vi "Main Page.vi"(8 "error in (no error)":errorcluster, 11 "Node Ptr":T2 format="%.0x") -> (0 "error out":errorcluster)   [LabVIEW 2017, in "OPC UA Client System Explorer.lvlib"]
uses:
  OPC UA Client System Explorer.lvlib
  <vilib>/NI Veristand/Custom Device API/Custom Device Item Ref.ctl
  Shared/OPCConnection.Properties.ctl
  Shared/Constants.vi
  <vilib>/NI Veristand/Custom Device API/NI VeriStand - Get Item Property.vi
  <vilib>/NI Veristand/Custom Device API/Get Item Property (String).vi
  <vilib>/NI Veristand/Custom Device API/Get Item Property (U16).vi
  <vilib>/NI Veristand/Custom Device API/Get Item Property (Dependent File).vi
  <vilib>/NI Veristand/Custom Device API/NI VeriStand - Set Item Property.vi
  <vilib>/NI Veristand/Custom Device API/Set Item Property (String).vi
  <vilib>/NI Veristand/Custom Device API/Set Item Property (U16).vi
  <vilib>/Utility/libraryn.llb/Get File Extension.vi
  <vilib>/Utility/MD5Checksum.llb/MD5Checksum File.vi
  <vilib>/NI Veristand/Custom Device API/Set Item Property (Dependent File).vi
  <vilib>/NI Veristand/Custom Device API/NI VeriStand - Remove Item Property.vi
  <vilib>/NI VeriStand/Custom Device API/Custom Device API.lvlib
  Shared/OPC UA Client Shared.lvlib
panel:
  in  "Header 2":cluster{"Section Name":string}={"Section Name"="Connection Settings"}
  in  "Login Info":cluster{"User Name":string, "Password":string}
  in  "Security Policy":T1
  in  "Server Certificate":path
  in  "Client Certificate":path
  in  "Server Port":u16=49350
  in  "Server IP Address":string
  in  "SHDocVw.IWebBrowser":refnum<k7>(container)
  in  "Header":cluster{"Section Name":string}={"Section Name"="Custom Device Item Settings"}
  in  "Description":string
  in  "Name":string
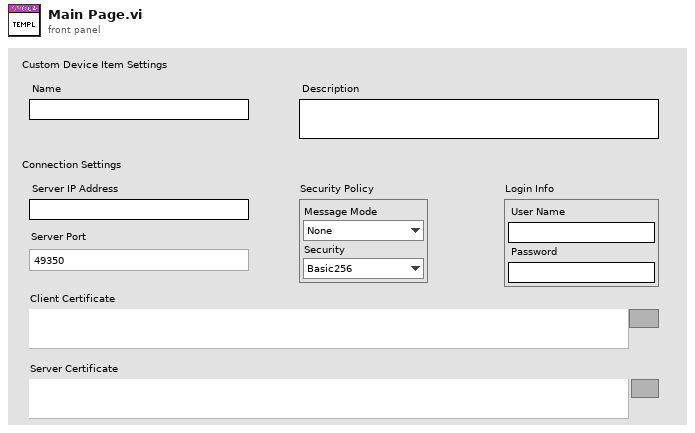
[diagram p1: front panel]
types:
  T1 = cluster{"Message Mode":enum16{"None", "Sign", "Sign and Encrypt"}, "Security":enum16{"Basic256", "Basic128Rsa15"}}
  T2 = typedef "Custom Device API.lvlib/Custom Device Item Ref.ctl" = u64
  T3 = typedef "Custom Device API.lvlib/Custom Device Item Info.ctl" = cluster{"Name":string, "Is Channel":bool, "GUID":string, "Is Waveform":bool}
  T4 = typedef "OPC UA Client Shared.lvlib/OPCConnection.Properties.ctl" = cluster{"Server IP Address":string, "Server Port":u16, "Message Mode":enum16{"None", "Sign", "Sign and Encrypt"}, "Security":enum16{"Basic256", "Basic128Rsa15"}, "User Name":string, "Password":string, "Client Certificate":path, "Server Certificate":path, "Server Certificate (RT)":path, "Client Certificate (RT)":path}
  T5 = typedef "Custom Device API.lvlib/Custom Device Commands.ctl" = enum16{"Default", "Item renamed", "Shutdown", "Dynamic button pressed"}
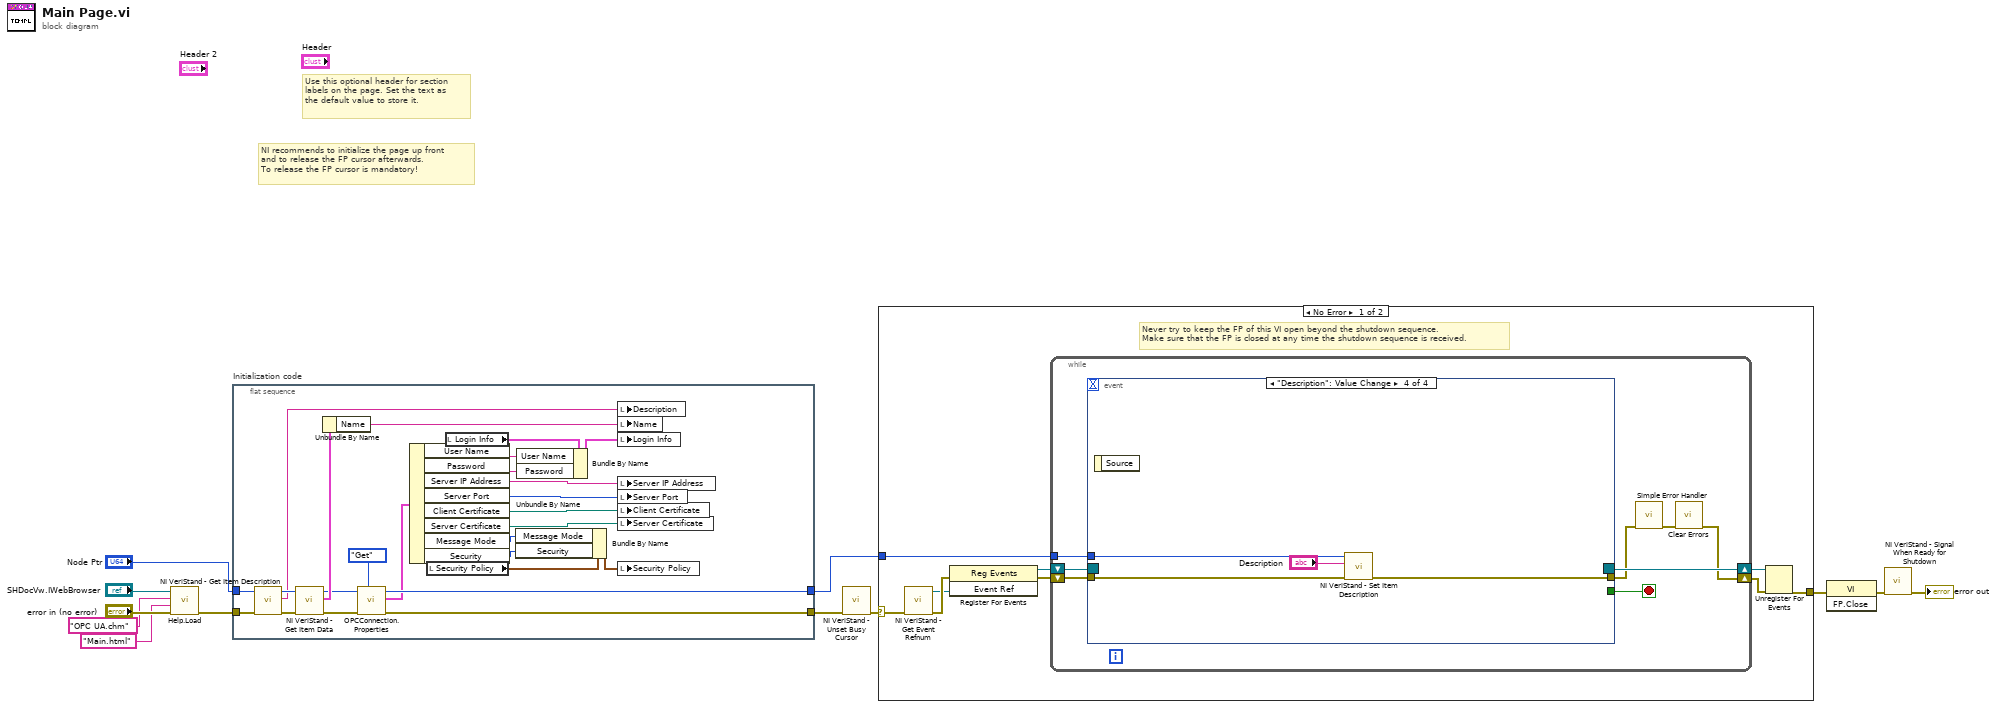
[diagram p0: block diagram]
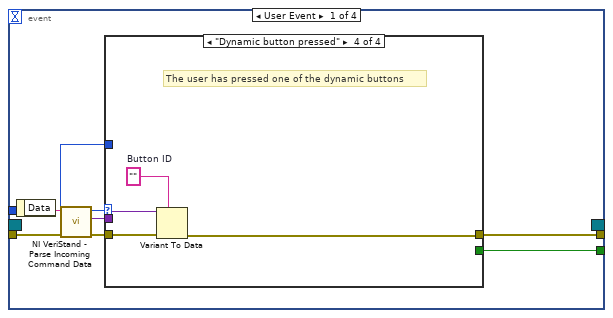
[diagram p2: hidden frame]
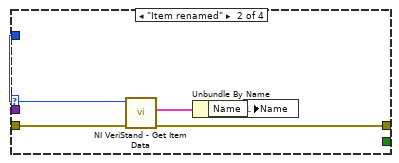
[diagram p4: hidden frame]
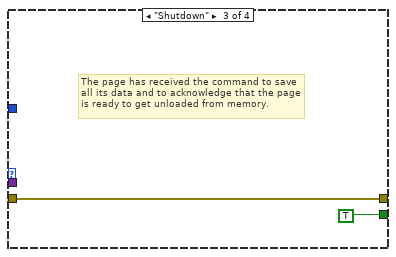
[diagram p5: hidden frame]
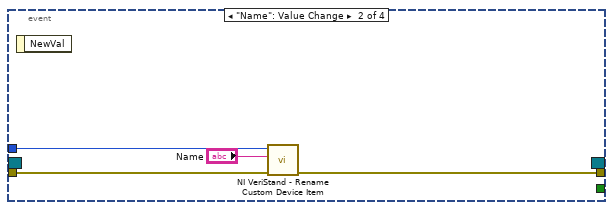
[diagram p6: hidden frame]
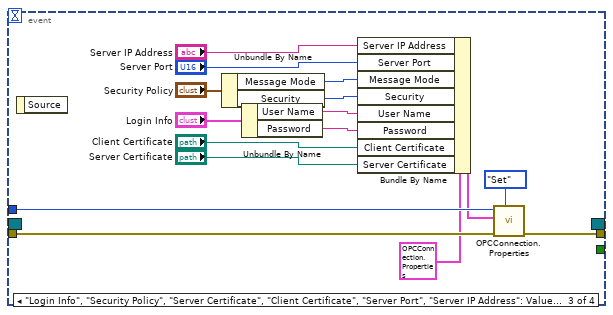
[diagram p7: hidden frame]
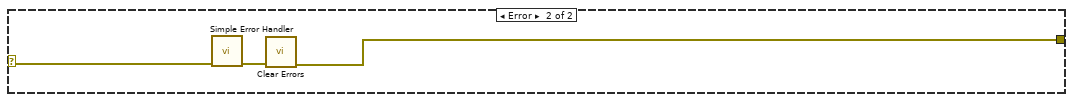
[diagram p8: hidden frame]
diagram:
  # "Use this optional header for section labels on the page. Set the text as the default value to store it."
  # "NI recommends to initialize the page up front\nand to release the FP cursor afterwards.\nTo release the FP cursor is mandatory!"
  n1 = call "Help.Load.vi"("error in (no error)"="error in (no error)", "HTML File"="Main.html" ("Main CHM File"), "Main CHM File"="OPC UA.chm", "SHDocVw.IWebBrowser2"="SHDocVw.IWebBrowser") -> ("error out"=w4:errorcluster)  [unwired: 7 in]
  n2 = flat-sequence "Initialization code" {
    tunnel: w4 -> [w36]
    tunnel: "Node Ptr" -> [w35]
    tunnel: [w28] -> w8
    tunnel: [w26] -> w6
    frame #0 {
      n3 = call <vilib>:"NI VeriStand - Get Item Description.vi"("error in (no error)"=w36, "Item Ref in"=w35) -> ("error out"=w33:errorcluster, "Description"=w34:string, "Item Ref out"=w37:T2)  [unwired: 7 out]
      n4 = call <vilib>:"NI VeriStand - Get Item Data.vi"("error in (no error)"=w33, "Item Ref in"=w37) -> ("error out"=w29:errorcluster, "Item Info"=w32:T3, "Item Ref out"=w27:T2)  [unwired: 7 out]
      n5 = Unbundle By Name(w32) -> ("Name"=w31:string)
      n6 = call "OPCConnection.Properties.vi"("Action"=enum8{"Get", "Set"}."Get", "error in (no error)"=w29, "Item Ref in"=w27) -> ("error out"=w28:errorcluster, "Connection.Properties"=w25:T4, "Item Ref out"=w26:T2)  [unwired: 6 in]
      n7 = Unbundle By Name(w25) -> ("User Name"=w23:string, "Password"=w22:string, "Server IP Address"=w20:string, "Server Port"=w19:u16, "Client Certificate"=w18:path, "Server Certificate"=w17:path, "Message Mode"=w14:enum16{"None", "Sign", "Sign and Encrypt"}, "Security"=w13:enum16{"Basic256", "Basic128Rsa15"})
      n8 = local read "Security Policy"() -> (w15:T1)
      n9 = local read "Login Info"() -> (w24:cluster{"User Name":string, "Password":string})
      n10 = Bundle By Name(cluster=w15, "Message Mode"=w14, "Security"=w13) -> (w16:T1)
      n11 = Bundle By Name(cluster=w24, "User Name"=w23, "Password"=w22) -> (w21:cluster{"User Name":string, "Password":string})
      n12 = local write "Description"(w34) -> ()
      n13 = local write "Name"(w31) -> ()
      n14 = local write "Login Info"(w21) -> ()
      n15 = local write "Server IP Address"(w20) -> ()
      n16 = local write "Server Port"(w19) -> ()
      n17 = local write "Client Certificate"(w18) -> ()
      n18 = local write "Server Certificate"(w17) -> ()
      n19 = local write "Security Policy"(w16) -> ()
    }
  }
  n20 = call <vilib>:"NI VeriStand - Unset Busy Cursor.vi"("error in (no error)"=w8) -> ("error out"=w7:errorcluster)  [unwired: 10 out]
  n21 = case shown="No Error" w7 {
    selector: w7 -> [w38 w101]
    tunnel: [w43 w99] -> w12
    tunnel: w6 -> [w39 _]
    frame No Error {
      # "Never try to keep the FP of this VI open beyond the shutdown sequence.\nMake sure that the FP is closed at any time the shutdown sequence is received."
      n22 = call <vilib>:"NI VeriStand - Get Event Refnum.vi"("error in (no error)"=w38) -> ("error out"=w46:errorcluster, "Event Ref"=w42:refnum<user-event>)  [unwired: 9 out]
      n23 = register-events(error in=w46, w42) -> (reference out=w40:refnum<event-registration>, error out=w41:errorcluster)  [unwired: 1 in]
      n24 = while {
        tunnel: w39 -> [w50]
        shift-right: [w47] -> w44
        shift-left: w41 -> [w53]
        shift-right: [w54] -> w45
        shift-left: w40 -> [w52]
        stop <- w51 stop-if-true
        n25 = event shown="[3] \"Description\": Value Change" {
          selector: w52 -> [_ _ _ _]
          dyn-events: [_ _ _ _] -> w54
          timeout: _ -> [_ _ _ _]
          tunnel: w53 -> [w62 w78 w93 w97]
          tunnel: [w58 _ _ _] -> w51
          tunnel: [w57 w77 w92 w96] -> w49
          tunnel: w50 -> [w56 w76 w91 w98]
          event User Event {
            n26 = event-data() -> ("Data"=w61:string)  [unwired: 1 out]
            n27 = call <vilib>:"NI VeriStand - Parse Incoming Command Data.vi"("error in (no error)"=w62, "Incoming data"=w61) -> ("error out"=w60:errorcluster, "Outgoing data"=w55:variant, "Action"=w59:T5)  [unwired: 7 out]
            n28 = case shown="\"Dynamic button pressed\"" w59 {
              tunnel: w60 -> [w63 w68 w69 w74]
              tunnel: [_ _ TRUE _] -> w58
              tunnel: [w63 w65 w69 w71] -> w57
              tunnel: w56 -> [_ w67 _ _]
              tunnel: w55 -> [_ _ _ w73]
              frame "Default", Default {
              }
              frame "Item renamed" {
                n29 = call <vilib>:"NI VeriStand - Get Item Data.vi"("error in (no error)"=w68, "Item Ref in"=w67) -> ("error out"=w65:errorcluster, "Item Info"=w66:T3)  [unwired: 8 out]
                n30 = Unbundle By Name(w66) -> ("Name"=w64:string)
                n31 = local write "Name"(w64) -> ()
              }
              frame "Shutdown" {
                # "The page has received the command to save all its data and to acknowledge that the page is ready to get unloaded from memory."
              }
              frame "Dynamic button pressed" {
                w72 = ""  # Button ID
                # "The user has pressed one of the dynamic buttons"
                n32 = Variant To Data(error in=w74, type=w72, Variant=w73) -> (error out=w71:errorcluster)  [unwired: 1 out]
              }
            }
          }
          event "Name": Value Change {
            n33 = event-data() -> ()  [unwired: 2 out]
            n34 = call <vilib>:"NI VeriStand - Rename Custom Device Item.vi"("error in (no error)"=w78, "New Name"="Name", "Item Ref in"=w76) -> ("error out"=w77:errorcluster)  [unwired: 1 in, 7 out]
          }
          event "Login Info", "Security Policy", "Server Certificate", "Client Certificate", "Server Port", "Server IP Address": Value Change {
            n35 = event-data() -> ()  [unwired: 2 out]
            n36 = Unbundle By Name("Security Policy") -> ("Message Mode"=w83:enum16{"None", "Sign", "Sign and Encrypt"}, "Security"=w82:enum16{"Basic256", "Basic128Rsa15"})
            n37 = Unbundle By Name("Login Info") -> ("User Name"=w86:string, "Password"=w85:string)
            n38 = Bundle By Name(cluster=T4 {"Server IP Address"="localhost", "Server Port"=49350, "Message Mode"=enum."None", "Security"=enum."Basic256", "User Name"="", "Password"="", "Client Certificate"=path "", "Server Certificate"=path "", "Server Certificate (RT)"=path "", "Client Certificate (RT)"=path ""} ("Connection.Properties"), "Server IP Address"="Server IP Address", "Server Port"="Server Port", "Message Mode"=w83, "Security"=w82, "User Name"=w86, "Password"=w85, "Client Certificate"="Client Certificate", "Server Certificate"="Server Certificate") -> (w79:T4)
            n39 = call "OPCConnection.Properties.vi"("Action"=enum8{"Get", "Set"}."Set", "error in (no error)"=w93, "Connection.Properties"=w79, "Item Ref in"=w91) -> ("error out"=w92:errorcluster)  [unwired: 5 in, 2 out]
          }
          event "Description": Value Change {
            n40 = event-data() -> ()  [unwired: 2 out]
            n41 = call <vilib>:"NI VeriStand - Set Item Description.vi"("error in (no error)"=w97, "Description"="Description", "Item Ref in"=w98) -> ("error out"=w96:errorcluster)  [unwired: 8 out]
          }
        }
        n42 = call <vilib>:"Simple Error Handler.vi"("error in (no error)"=w49) -> ("error out"=w48:errorcluster)  [unwired: 1 in, 7 out]
        n43 = call <vilib>:"Clear Errors.vi"("error in (no error)"=w48) -> ("error out"=w47:errorcluster)  [unwired: 1 in, 5 out]
      }
      n44 = Unregister For Events(event registration refnum=w45, error in=w44) -> (error out=w43:errorcluster)
    }
    frame Error {
      n45 = call <vilib>:"Simple Error Handler.vi"("error in (no error)"=w101) -> ("error out"=w100:errorcluster)  [unwired: 1 in, 7 out]
      n46 = call <vilib>:"Clear Errors.vi"("error in (no error)"=w100) -> ("error out"=w99:errorcluster)  [unwired: 1 in, 5 out]
    }
  }
  n47 = invoke class="VI" method="FP.Close"(error in=w12) -> (error out=w11:errorcluster)  [unwired: 2 in, 2 out]
  n48 = call <vilib>:"NI VeriStand - Signal When Ready for Shutdown.vi"("error in (no error)"=w11) -> ("error out"=→"error out":errorcluster)  [unwired: 10 out]
